vi "WS1033_Multi-socket save data ver1.0.vi"(0 "TMN DC\\CAP Data Log File Path":path=path "C:/temp", 1 "TP/Comment":cluster{"Test Program":string, "Comment":string}={"Test Program"="Multi Socket", "Comment"="HD_Cycling"}, 2 "Data Output Reg1&2":string[][](table), 3 "SN":string[](array[string]), 4 "HD/Cycles Completed":string="Test Data", 5 "Lot#":string="WS1033", 6 "Data Output Reg3&4":string[][](table), 7 "Wafer#":string="T4", 8 "Current":string[](array[string]), 9 "File Name":string="Test Data", 10 "VPI Out":string[][](array[string]), 11 "error in":errorcluster, 12 "EFuse":string[](array[string])=["0A", "0A", "0A", "0A", "0A", "0A", "0A", "0A", "0A", "0A", "0A", "0A", "0A", "0A", "0A", "0A"], 13 "Bin":string[](array[string])=["0A", "0A", "0A", "0A", "0A", "0A", "0A", "0A", "0A", "0A", "0A", "0A", "0A", "0A", "0A", "0A"], 14 "R/W Status":string[](array[string])=["PASS", "PASS", "PASS", "PASS", "PASS", "PASS", "PASS", "PASS", "PASS", "PASS", "PASS", "PASS", "PASS", "PASS", "PASS", "PASS"]) -> (15 "error out":errorcluster)   [LabVIEW 2012]
panel:
  in  "Output":string[][](table)
  # "**************** Do Not Remove *******\nCompany:  WiSpry Inc\n20 Fairbanks Ste 198 Irvine CA 92618\n\nAuthor:  Andy V Tran\nCreated:  03/06/2013\nLabVIEW 2009 Pro\nTP:  Multi-Socket Save Data ver1.0\n*******************************************"
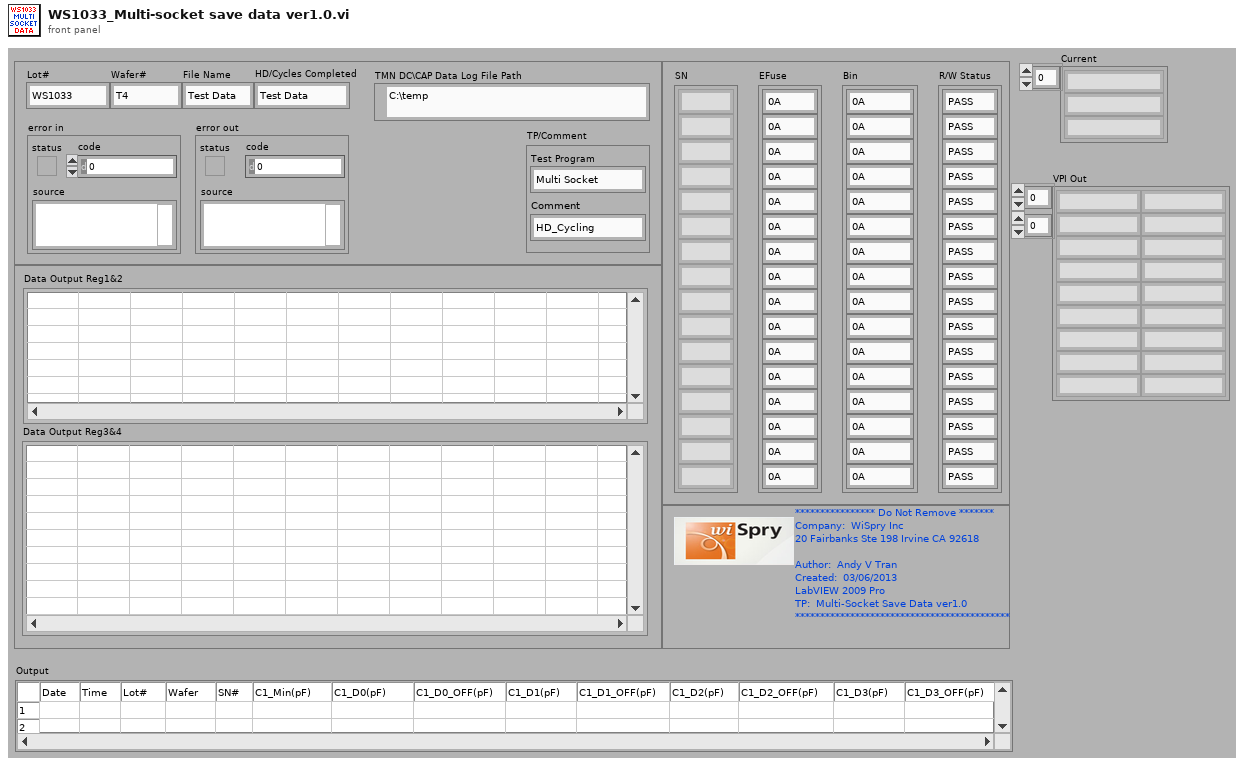
[diagram p1: front panel]
types:
  T1 = enum16{"open", "replace", "create", "open or create", "replace or create", "replace or create with confirmation"}
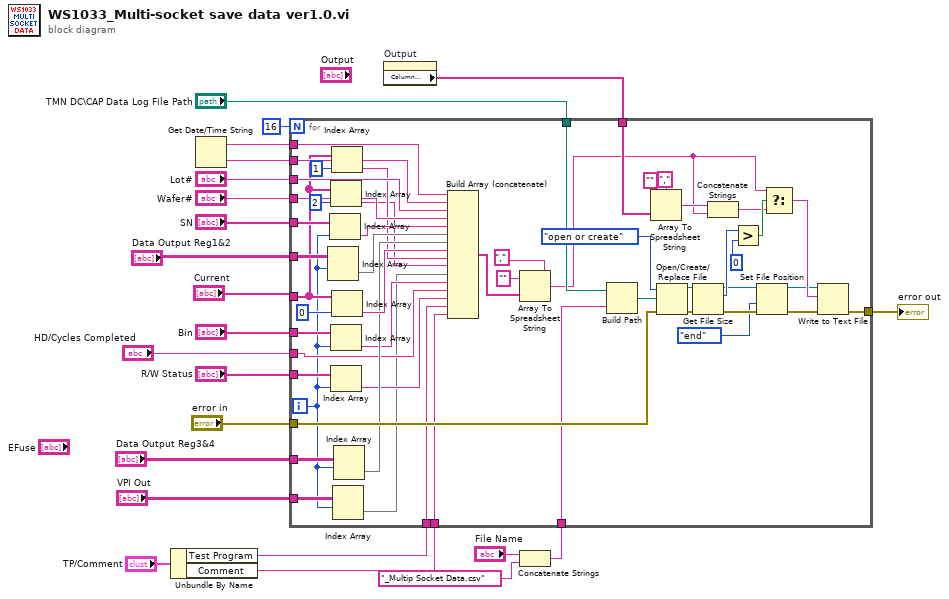
[diagram p0: block diagram]
diagram:
  n1 = Unbundle By Name("TP/Comment") -> ("Test Program"=w13:string, "Comment"=w12:string)
  n2 = Get Date/Time String() -> (date string=w7:string, time string=w8:string)  [unwired: 3 in]
  n3 = property on="Output" class="Tbl (strict)"() -> ("Column Headers[]"=w22:string[])  [unwired: 2 in, 2 out]
  n4 = Concatenate Strings("File Name", "_Multip Socket Data.csv" ("string")) -> (w16:string)
  n5 = for {
    N: 16 -> [_]
    tunnel: "TMN DC\\CAP Data Log File Path" -> [w76]
    tunnel: w22 -> [w75]
    tunnel: "Wafer#" -> [w74]
    tunnel: "error in" -> [w73]
    tunnel: w16 -> [w72]
    tunnel: [w50] -> w15
    tunnel: "SN" -> [w49]
    tunnel: "Current" -> [w34]
    tunnel: w13 -> [w30]
    tunnel: w12 -> [w31]
    tunnel: "Bin" -> [w47]
    tunnel: "R/W Status" -> [w46]
    tunnel: "Lot#" -> [w45]
    tunnel: w8 -> [w44]
    tunnel: w7 -> [w43]
    tunnel: "HD/Cycles Completed" -> [w28]
    tunnel: "Data Output Reg1&2" -> [w41]
    tunnel: "Data Output Reg3&4" -> [w39]
    tunnel: "VPI Out" -> [w26]
    i -> [w24]
    n6 = Index Array(array=w41, index (row)=w24) -> (element=w40:string[])  [unwired: 1 in]
    n7 = Index Array(array=w49, index=w24) -> (element=w48:string)
    n8 = Index Array(array=w34, index=2) -> (element=w32:string)
    n9 = Index Array(array=w47, index=w24) -> (element=w27:string)
    n10 = Index Array(array=w46, index=w24) -> (element=w29:string)
    n11 = Index Array(array=w34, index=1) -> (element=w33:string)
    n12 = Index Array(array=w34, index=0) -> (element=w42:string)
    n13 = Index Array(array=w26, index (row)=w24) -> (element=w25:string[])  [unwired: 1 in]
    n14 = Index Array(array=w39, index (row)=w24) -> (element=w38:string[])  [unwired: 1 in]
    n15 = Build Array (concatenate)(w43, w44, w45, w74, w48, w40, w38, w42, w33, w32, w25, w27, w28, w29, w30, w31) -> (w51:string[])
    n16 = Array To Spreadsheet String(delimiter (Tab)=",", array=w51, 3:"" ("format string")) -> (spreadsheet string=w52:string)
    n17 = Build Path(base path=w76, name or relative path=w72) -> (appended path=w66:path)
    n18 = Array To Spreadsheet String(delimiter (Tab)=",", array=w75, 3:"" ("format string")) -> (spreadsheet string=w54:string)
    n19 = Open/Create/Replace File(file path (use dialog)=w66, error in=w73, operation (0:open)=T1."open or create") -> (refnum out=w64:refnum<file>, error out=w67:errorcluster)  [unwired: 4 out]
    n20 = Get File Size(file=w64, error in=w67) -> (refnum out=w59:refnum<file>, size (in bytes)=w63:i64, 0:w61:errorcluster)
    n21 = Concatenate Strings(w54, w52) -> (w53:string)
    n22 = Greater?(x=w63, y=i64 0) -> (0:w68:bool)
    n23 = Set File Position(refnum=w59, from (0:start)=enum16{"start", "end", "current"}."end", error in=w61) -> (refnum out=w58:refnum<file>, error out=w60:errorcluster)  [unwired: 1 out]
    n24 = Select(t=w52, s=w68, f=w53) -> (s? t:f=w65:string)
    n25 = Write to Text File(file (use dialog)=w58, text=w65, error in=w60) -> (error out=w50:errorcluster)  [unwired: 3 out]
  }
  "error out" <- w15
